vi "Measure AC Parameters.vi"(6 "maximum harmonic":i32=5, 8 "error in":errorcluster, 9 "Full scale range":dbl=5.0 format="%#_13g", 11 "Acquired waveform":waveform(dbl)) -> (0 "error out":errorcluster, 2 "Single tone results":T1, 3 "FFT":cluster{"x0":dbl, "dx":dbl, "magnitude":dbl[]} {"magnitude" format="%.2p"; "dx" format="%.2p"; "x0" format="%.2p"})   [LabVIEW 2021, in "Single Tone_DAC.lvlib"]
uses:
  Single Tone_DAC.lvlib
  <vilib>/addons/_NISVFA/_Shared subVIs/Controls/svc_Window.ctl
  <vilib>/addons/_NISVFA/_Shared subVIs/Common/SVL Set dB Reference (1 Ch).vi
  <vilib>/addons/_NISVFA/_Spectrum Processing/SVFA Get Spectrum Subset (Complex) (1 Ch).vi
  <vilib>/addons/Sound and Vibration/svt_Single Tone Measurements/SVT Spurious Free Dynamic Range (Frequency) (1 Ch).vi
  <vilib>/addons/_NISVFA/_Spectrum Processing/SVFA Unit Conversion (Complex) (1 Ch).vi
  <vilib>/addons/_NISVFA/_Shared subVIs/Common/SVL Set dB Reference (variant).vi
  <vilib>/addons/_NISVFA/_Shared subVIs/Common/svc_Check Frequency Range in Spectrum.vi
  <vilib>/addons/_NISVFA/_Shared subVIs/Common/svc_Build Unit Label for Frequency Range.vi
  <vilib>/addons/_NISVFA/_Shared subVIs/Common/svc_Window Parameters.vi
  <vilib>/addons/_NISVFA/_Shared subVIs/Common/svc_Extract Single Tone Information (complex).vi
  <vilib>/addons/_NISVFA/_Spectrum Processing/SVFA Spectrum Peak Search.vi
  <vilib>/addons/_NISVFA/_Spectrum Processing/SVFA Spectrum Peak Search (1 Ch).vi
  <vilib>/addons/_NISVFA/_Shared subVIs/Common/svc_Spectrum Units.vi
  <vilib>/addons/_NISVFA/_Shared subVIs/Common/svc_Log View for Spectrum (1Ch).vi
  <vilib>/addons/_NISVFA/_Spectrum Processing/SVFA Unit Conversion (1 Ch).vi
  <vilib>/addons/_NISVFA/_Shared subVIs/Common/svc_Complex Datatype Defaults.vi
  <vilib>/addons/_NISVFA/_Shared subVIs/Common/svc_Check Frequency Range in Bandwidth.vi
  <vilib>/addons/_NISVFA/_Shared subVIs/Common/svc_Convert Start and Stop to Start Index and Length.vi
  <vilib>/addons/_NISVFA/_Spectrum Processing/SVFA Get Tone Amplitude and Phase (1 Ch).vi
  <vilib>/addons/_NISVFA/_Spectrum Processing/subVIs/svfa_Compute Complex Spectrum for Export.vi
  <vilib>/addons/_NISVFA/_Spectrum Processing/subVIs/svfa_Spectrum Peak Search.vi
  <vilib>/addons/_NISVFA/_Shared subVIs/Common/svc_Format Value (DBL).vi
  <vilib>/addons/_NISVFA/_Shared subVIs/Common/svc_Get Weighting Enum and Labels.vi
  <vilib>/addons/_NISVFA/_Shared subVIs/Common/svc_Engineering Units to Unit Label.vi
  <vilib>/addons/_NISVFA/_Shared subVIs/Common/svc_Surround NonAlpha String with Parentheses.vi
  <vilib>/dlg_ctls.llb/Space Constant.vi
  <vilib>/addons/_NISVFA/_Shared subVIs/Common/svc_Unwrap Phase.vi
  <vilib>/addons/_NISVFA/_Shared subVIs/Common/svc_Convert Spectrum Array to dB.vi
  <vilib>/addons/_NISVFA/_Spectrum Processing/subVIs/svfa_Conversion Utility (spectrum info).vi
  <vilib>/addons/_NISVFA/_Spectrum Processing/subVIs/svfa_Window Frequency Response.vi
  <vilib>/addons/_NISVFA/_Spectrum Processing/subVIs/svfa_Window Frequency Response (double array).vi
  <vilib>/Analysis/baseanly.llb/Dot Product.vi
  <vilib>/Analysis/baseanly.llb/Complex Dot Product.vi
  <vilib>/addons/_NISVFA/_Spectrum Processing/subVIs/svfa_Peak Rough Search Indices.vi
  <vilib>/addons/_NISVFA/_Shared subVIs/Common/svc_Unit Label Lexical Class.vi
  <vilib>/addons/_NISVFA/_Spectrum Processing/subVIs/svfa_Peak to RMS to Peak2Peak.vi
  <vilib>/addons/_NISVFA/_Spectrum Processing/subVIs/svfa_Mag to Mag2.vi
  <vilib>/addons/_NISVFA/_Spectrum Processing/subVIs/svfa_Linear to dB.vi
  <vilib>/addons/_NISVFA/_Spectrum Processing/subVIs/svfa_dBrefA to dBrefB.vi
  <vilib>/addons/_NISVFA/_Spectrum Processing/subVIs/svfa_Spectrum to Spectral Density.vi
  <vilib>/addons/_NISVFA/_Spectrum Processing/subVIs/svfa_Rect Window Frequency Response.vi
  <vilib>/addons/_NISVFA/_Spectrum Processing/subVIs/svfa_Cosine Window Coefficients.vi
  <vilib>/addons/_NISVFA/_Shared subVIs/Common/svc_Caller VI Returned in Error Source.vi
  <vilib>/addons/_NISVFA/_Baseband FFT/SVFA FFT Spectrum (Complex) (1 Ch).vi
  <vilib>/addons/_NISVFA/_Shared subVIs/Common/svc_Convert Frequency to Frequency String.vi
  <vilib>/addons/Sound and Vibration/svt_Distortion/SVT SNR without Harmonics (Frequency) (1 Ch).vi
  <vilib>/addons/Sound and Vibration/svt_Distortion/subVIs/sv_Check Data Valid (Audio) (1 Ch).vi
  <vilib>/Analysis/4window.llb/window parameters.vi
  <vilib>/Analysis/4window.llb/Window Properties.vi
  <vilib>/Analysis/4window.llb/Window Properties by Name.vi
  <vilib>/addons/_NISVFA/_Spectrum Processing/subVIs/svfa_Spectrum Peak Tone Search and Estimation (complex).vi
  <vilib>/measure/masignal.llb/Tones and Noise Waveform.vi
  <vilib>/addons/_NISVFA/_Shared subVIs/Common/svc_FFT with Window.vi
  <vilib>/Analysis/1siggen.llb/Square Wave.vi
  <vilib>/addons/_NISVFA/_Spectrum Processing/subVIs/svfa_Three Finger Peak Search.vi
  <vilib>/addons/Sound and Vibration/svt_Distortion/subVIs/sv_Peak View Amplitude (1 Ch).vi
  <vilib>/addons/Sound and Vibration/svt_Distortion/SoundVib_Distortion.lvlib
  <vilib>/addons/Sound and Vibration/svt_Single Tone Measurements/SoundVib_SingleTone.lvlib
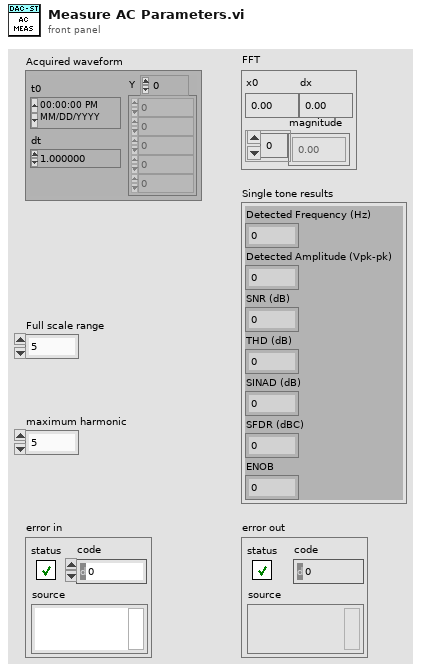
[diagram p1: front panel]
types:
  T1 = cluster{"Detected Frequency (Hz)":dbl, "Detected Amplitude (Vpk-pk)":dbl, "SNR (dB)":dbl, "THD (dB)":dbl, "SINAD (dB)":dbl, "SFDR (dBC)":dbl, "ENOB":dbl}
  T2 = typedef "svc_Window.ctl" = u32
  T3 = enum16{"no change", "spectrum", "spectral density"}
  T4 = cluster{"SNR units":enum16{"dB", "linear ratio", "%"}, "detected fundamental amplitude units":enum16{"EU rms", "EU peak", "EU peak-peak"}}
  T5 = cluster{"linear/dB":enum16{"no change", "linear", "dB"}, "dB reference (0: no change)":dbl, "power/magnitude":enum16{"no change", "power", "magnitude"}, "view":enum16{"no change", "rms", "peak", "peak-peak"}}
  T6 = typedef "svc_Spectrum Info.ctl" = cluster{"channel name":string, "description":string, "x-axis units":T7, "spectral info":cluster{"spectrum type":T8, "linear/dB":enum16{"linear", "dB"}, "window":u16, "window size":i32, "FFT size":i32}, "engineering units":T9, "custom label":string, "dB reference [EU]":dbl, "peak units":enum16{"rms", "peak", "peak-peak"}, "weighting filter":T10, "spectral density?":bool, "unit label":string, "spectrum skewed?":bool, "complimentary spectrum units":T11}
  T7 = typedef "svc_X-Axis Units.ctl" = u16
  T8 = typedef "svc_Spectrum Type.ctl" = enum16{"FFT Spectrum [complex]", "Amplitude [Magnitude]", "Power [Magnitude^2]", "Cross Spectrum [complex]", "Frequency Response [Complex]"}
  T9 = typedef "svc_Engineering Units Text Ring.ctl" = u16
  T10 = typedef "svc_Weighting Filter Text Ring.ctl" = u16
  T11 = typedef "svc_Complimentary Spectrum Units.ctl" = enum16{"none", "radians", "degrees", "cycles", "imaginary"}
  T12 = cluster{"complex spectrum response":cluster{"f0":dbl, "df":dbl, "complex spectrum":cdb[]}, "spectrum info":T6}
  T13 = cluster{"complex spectrum subset":cluster{"x0":dbl, "dx":dbl, "complex array":cdb[]}, "spectrum info":T6}
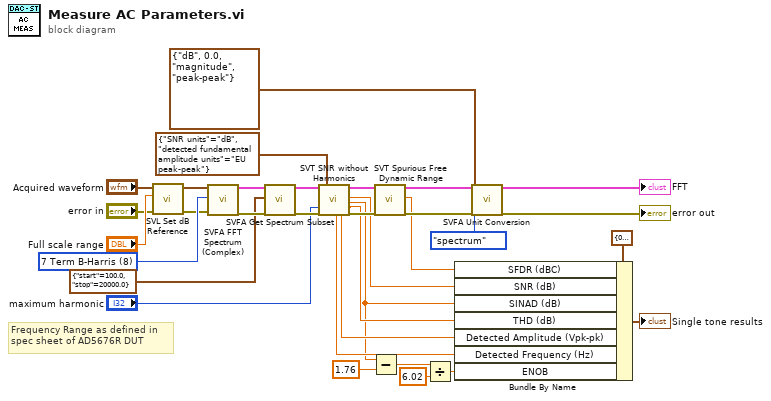
[diagram p0: block diagram]
diagram:
  w33 = T2 8 items=["None"=0, "Hanning"=1, "Hamming"=2, "Blackman-Harris"=3, "Exact Blackman"=4, "Blackman"=5, "Flat Top"=6, "4 Term B-Harris "=7, "7 Term B-Harris"=8, "Low Sidelobe"=9, "Force"=64, "Exponential"=65, "Blackman Nuttall"=11, "Triangle"=30, "Bartlett-Hanning"=31, "Bohman"=32, "Parzen"=33, "Welch"=34, "Kaiser"=60, "Dolph-Chebyshev"=61, "Gaussian"=62] ("window")
  # "Frequency Range as defined in\nspec sheet of AD5676R DUT"
  n1 = call-poly <vilib>:"SVL Set dB Reference.vi"("error in (no error)"="error in", "dB reference [EU]"="Full scale range", "scaled signal in [EU]"="Acquired waveform") -> ("error out"=w18:errorcluster, "scaled signal out [EU]"=w22:waveform(dbl))  [unwired: 7 in]
  n2 = call-poly <vilib>:"SVFA FFT Spectrum (Complex).vi"("scaled signal [EU]"=w22, "window"=w33, "error in"=w18) -> ("complex spectrum"=w25:T12, "error out"=w32:errorcluster)  [unwired: 13 in, 2 out]
  n3 = call-poly <vilib>:"SVFA Get Spectrum Subset.vi"("complex spectrum"=w25, "range"=cluster{"start":dbl, "stop":dbl} {"start"=100.0, "stop"=20000.0}, "error in (no error)"=w32) -> ("complex spectrum subset"=w20:T13, "error out"=w30:errorcluster)  [unwired: 13 in, 2 out]
  n4 = call-poly <vilib>:"SVT SNR without Harmonics.vi"("complex spectrum"=w20, "maximum harmonic"="maximum harmonic", "error in (no error)"=w30, "desired units"=T4 {"SNR units"=enum."dB", "detected fundamental amplitude units"=enum."EU peak-peak"}) -> ("detected fundamental\nfrequency [Hz]"=w5:dbl, "detected fundamental\namplitude"=w4:dbl, "complex spectrum"=w17:T12, "SNR (without harmonics)"=w2:dbl, "SINAD"=w1:dbl, "THD"=w3:dbl, "error out"=w15:errorcluster)  [unwired: 8 in, 1 out]
  n5 = Subtract(x=w1, y=1.76) -> (x-y=w12:dbl)
  n6 = call-poly <vilib>:"SVT Spurious Free Dynamic Range.vi"("complex spectrum"=w17, "error in (no error)"=w15) -> ("complex spectrum"=w16:T12, "spurious free dynamic range"=w6:dbl, "error out"=w14:errorcluster)  [unwired: 10 in, 5 out]
  n7 = Divide(x=w12, y=6.02) -> (x/y=w9:dbl)
  n8 = Bundle By Name(cluster=T1 {"Detected Frequency (Hz)"=0.0, "Detected Amplitude (Vpk-pk)"=0.0, "SNR (dB)"=0.0, "THD (dB)"=0.0, "SINAD (dB)"=0.0, "SFDR (dBC)"=0.0, "ENOB"=0.0} ("Single tone results"), "SFDR (dBC)"=w6, "SNR (dB)"=w2, "SINAD (dB)"=w1, "THD (dB)"=w3, "Detected Amplitude (Vpk-pk)"=w4, "Detected Frequency (Hz)"=w5, "ENOB"=w9) -> (→"Single tone results":T1)
  n9 = call-poly <vilib>:"SVFA Unit Conversion.vi"("complex spectrum"=w16, "desired scaling"=T5 {"linear/dB"=enum."dB", "dB reference (0: no change)"=0.0, "power/magnitude"=enum."magnitude", "view"=enum."peak-peak"}, "spectral density desired"=T3."spectrum", "error in (no error)"=w14) -> ("converted spectrum"=→"FFT":cluster{"x0":dbl, "dx":dbl, "magnitude":dbl[]}, "error out"=→"error out":errorcluster)  [unwired: 10 in, 4 out]
